vi "convert wrist angle.vi"(10 "Horizontal Encoder Ct":dbl, 11 "Angle In":dbl) -> (2 "Angle Out":dbl, 3 "Encoder Count Out":dbl)   [LabVIEW 2018]
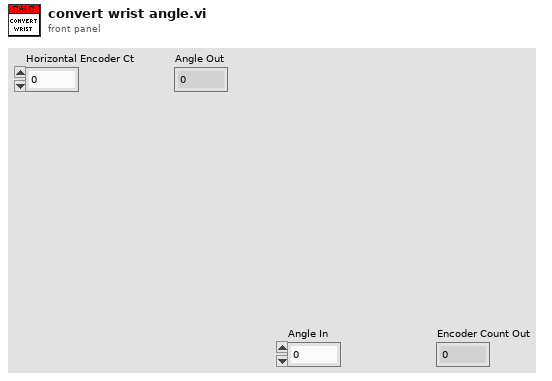
[diagram p1: front panel]
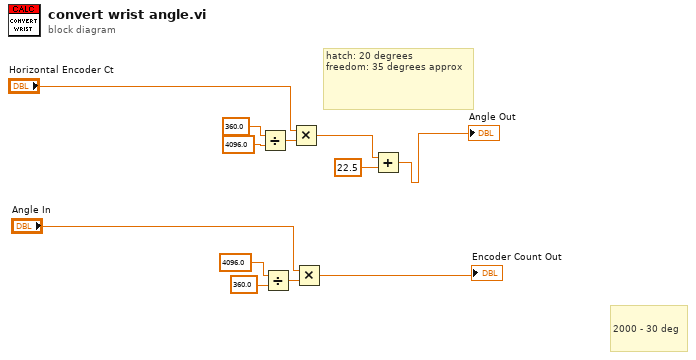
[diagram p0: block diagram]
diagram:
  # "hatch: 20 degrees\nfreedom: 35 degrees approx"
  # "2000 - 30 deg"
  n1 = Divide(x=360.0, y=4096.0) -> (x/y=w12:dbl)
  n2 = Divide(x=4096.0, y=360.0) -> (x/y=w8:dbl)
  n3 = Multiply(x="Horizontal Encoder Ct", y=w12) -> (x*y=w2:dbl)
  n4 = Multiply(x="Angle In", y=w8) -> (x*y=→"Encoder Count Out":dbl)
  n5 = Add(x=w2, y=22.5) -> (x+y=→"Angle Out":dbl)
